vi "Test_RTC.vi"(8 "error in (no error)":errorcluster, 10 "Parameters":string, 11 "reference in":refnum<class "Test_Flux_Capacitor.lvclass">) -> (0 "error out":errorcluster, 2 "Result":bool, 3 "reference out":refnum<class "Test_Flux_Capacitor.lvclass">)   [LabVIEW 2022 SP3, in "Test_Flux_Capacitor.lvlib" / "Test_Flux_Capacitor.lvclass"]
uses:
  Test_Flux_Capacitor.lvclass
  ParameterTypes/RTC.ctl
  Components/SwitchBase.lvlibp/SwitchBase.lvclass
  Components/PSU_Base.lvlibp/PSU_Base.lvclass
  Components/Flux_Capacitor.lvlibp/Flux_Capacitor.lvclass
  <vilib>/JDP Science/JSONtext/JSONtext.lvlib
panel:
  in  "Parameter_Type":T1
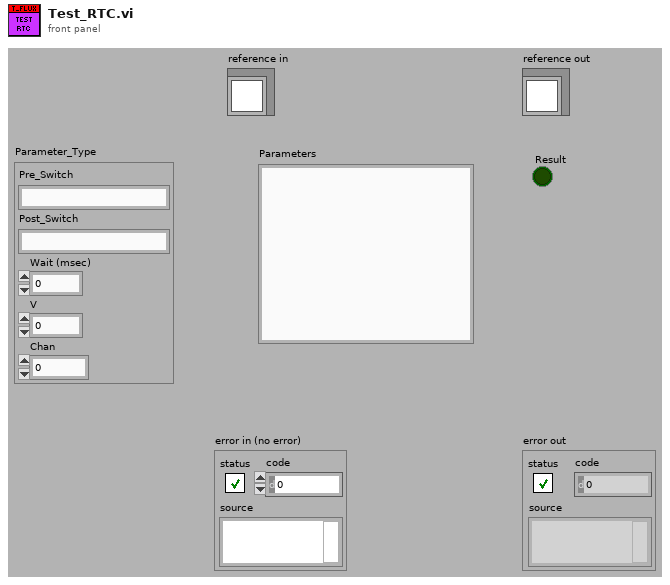
[diagram p1: front panel]
types:
  T1 = typedef "Test_Flux_Capacitor.lvlib/Test_Flux_Capacitor.lvclass/RTC.ctl" = cluster{"Pre_Switch":string, "Post_Switch":string, "Wait (msec)":u32, "V":dbl, "Chan":i32}
  T2 = typedef "Test_Flux_Capacitor.lvlib/Test_Flux_Capacitor.lvclass/ObjectAttributes.ctl" = cluster{"Config":T3, "DMM":refnum<class "DMM_Keysight_34980A.lvclass">, "LCR":refnum<class "LCR_BK891.lvclass">, "PSU":refnum<class "PSU_Base.lvclass">, "Switch_Manager":refnum<class "SwitchBase.lvclass">, "FRAM":string, "Flux_Capacitor":refnum<class "Flux_Capacitor.lvclass">, "Frequency_Counter":refnum<class "Frequency_Counter_Base.lvclass">, "JTAG":refnum<class "JTAG_Base.lvclass">}
  T3 = typedef "Test_Flux_Capacitor.lvlib/Test_Flux_Capacitor.lvclass/Config.ctl" = cluster{"default":string}
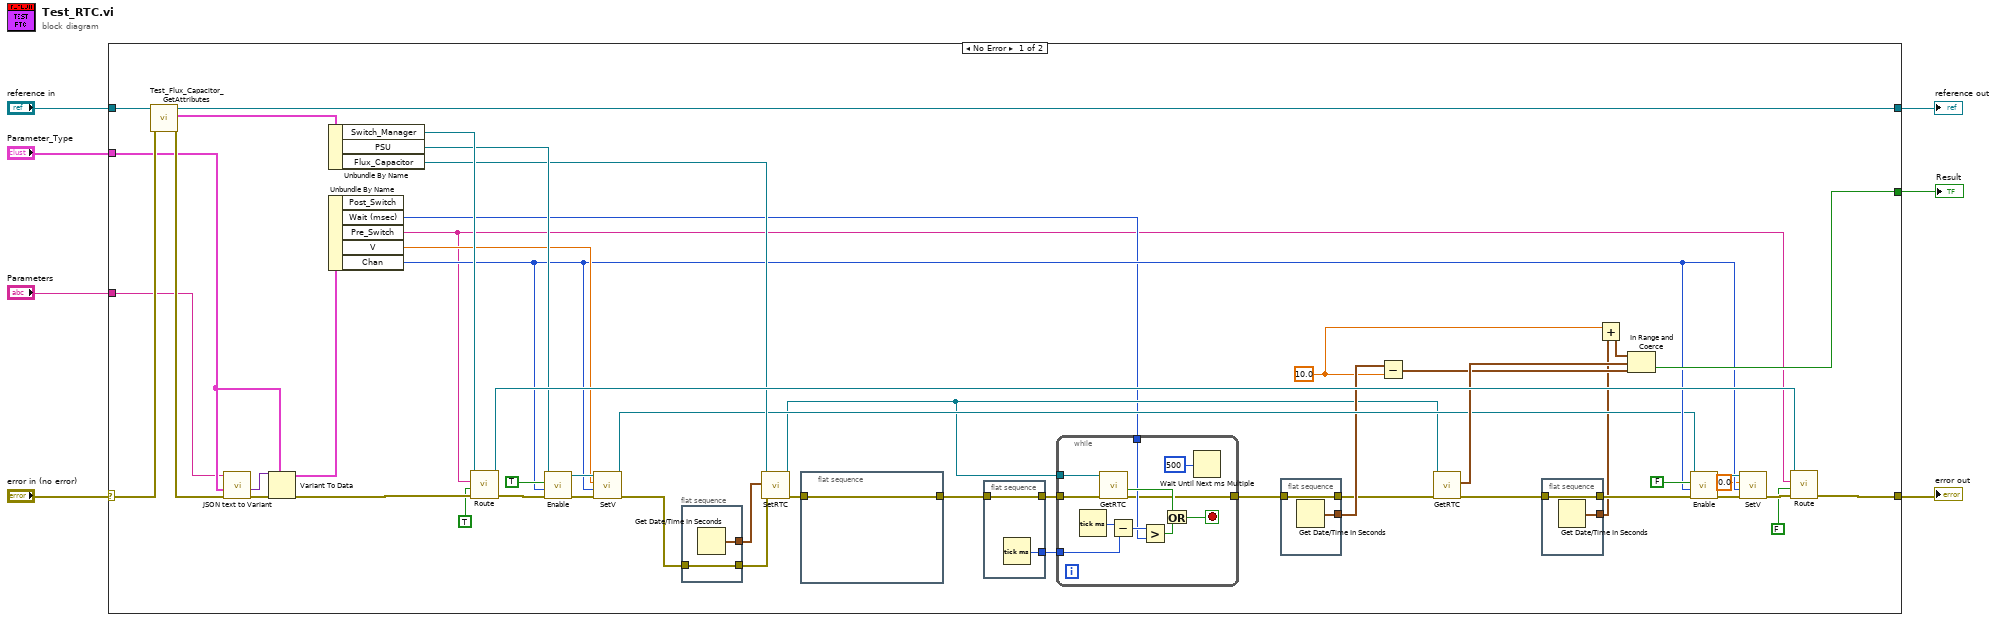
[diagram p0: block diagram]
diagram:
  n1 = case shown="No Error" "error in (no error)" {
    selector: "error in (no error)" -> [w58 w80]
    tunnel: [w51 w80] -> w6
    tunnel: [w56 w79] -> w4
    tunnel: "reference in" -> [w57 w79]
    tunnel: "Parameters" -> [w12 _]
    tunnel: "Parameter_Type" -> [w13 _]
    tunnel: [w38 _] -> w1
    frame No Error {
      w26 = 10.0
      n2 = call "Test_Flux_Capacitor_GetAttributes.vi"("error in (no error)"=w58, "reference in"=w57) -> ("error out"=w15:errorcluster, "Data"=w55:T2, "reference out"=w56:refnum<class "Test_Flux_Capacitor.lvclass">)  [unwired: 6 in, 1 out]
      n3 = call <vilib>:"JSON text to Variant.vi"("error in (no error)"=w15, "Data Type"=w13, "JSON"=w12) -> ("error out"=w14:errorcluster, "Variant out"=w11:variant)  [unwired: 7 in]
      n4 = Variant To Data(error in=w14, type=w13, Variant=w11) -> (data=w54:T1, error out=w50:errorcluster)
      n5 = Unbundle By Name(w55) -> ("Switch_Manager"=w53:refnum<class "SwitchBase.lvclass">, "PSU"=w47:refnum<class "PSU_Base.lvclass">, "Flux_Capacitor"=w43:refnum<class "Flux_Capacitor.lvclass">)
      n6 = Unbundle By Name(w54) -> ("Wait (msec)"=w16:u32, "Pre_Switch"=w9:string, "V"=w45:dbl, "Chan"=w31:i32)  [unwired: 1 out]
      n7 = call-dynamic "Route.vi"("error in (no error)"=w50, "Connect"=TRUE ("Enable"), "channel 1"=w9, "reference in"=w53) -> ("error out"=w49:errorcluster, "reference in"=w52:refnum<class "SwitchBase.lvclass">)  [unwired: 6 in]
      n8 = call-dynamic "Enable.vi"("error in (no error)"=w49, "Chan"=w31, "Enable"=TRUE, "reference in"=w47) -> ("error out"=w48:errorcluster, "reference in"=w46:refnum<class "PSU_Base.lvclass">)  [unwired: 6 in]
      n9 = call-dynamic "SetV.vi"("error in (no error)"=w48, "Chan"=w31, "V"=w45, "reference in"=w46) -> ("error out"=w32:errorcluster, "reference in"=w30:refnum<class "PSU_Base.lvclass">)  [unwired: 6 in]
      n10 = flat-sequence {
        tunnel: w32 -> [w78]
        tunnel: [w78] -> w42
        tunnel: [w77] -> w41
        frame #0 {
          n11 = Get Date/Time In Seconds() -> (seconds since 1Jan1904=w77:timestamp)
        }
      }
      n12 = call-dynamic "SetRTC.vi"("error in (no error)"=w42, "RTC"=w41, "reference in"=w43) -> ("error out"=w40:errorcluster, "reference in"=w20:refnum<class "Flux_Capacitor.lvclass">)  [unwired: 6 in, 1 out]
      n13 = flat-sequence {
        tunnel: w40 -> [w76]
        tunnel: [w76] -> w19
        frame #0 {
        }
      }
      n14 = flat-sequence {
        tunnel: w19 -> [w60]
        tunnel: [w60] -> w18
        tunnel: [w59] -> w17
        frame #0 {
          n15 = Tick Count (ms)() -> (millisecond timer value=w59:u32)
        }
      }
      n16 = while {
        tunnel: w18 -> [w70]
        tunnel: [w61] -> w21
        tunnel: w20 -> [w71]
        tunnel: w17 -> [w68]
        tunnel: w16 -> [w62]
        stop <- w64 stop-if-true
        n17 = Tick Count (ms)() -> (millisecond timer value=w69:u32)
        n18 = call-dynamic "GetRTC.vi"("error in (no error)"=w70, "reference in"=w71) -> ("error out"=w61:errorcluster, "OK"=w66:bool)  [unwired: 6 in, 2 out]
        n19 = Subtract(x=w69, y=w68) -> (x-y=w67:u32)
        n20 = Greater?(x=w67, y=w62) -> (0:w65:bool)
        n21 = Or(x=w66, y=w65) -> (x .or. y?=w64:bool)
        n22 = Wait Until Next ms Multiple(millisecond multiple=u32 500) -> ()  [unwired: 1 out]
      }
      n23 = flat-sequence {
        tunnel: [w75] -> w28
        tunnel: w21 -> [w74]
        tunnel: [w74] -> w22
        frame #0 {
          n24 = Get Date/Time In Seconds() -> (seconds since 1Jan1904=w75:timestamp)
        }
      }
      n25 = Subtract(x=w28, y=w26) -> (x-y=w27:timestamp)
      n26 = call-dynamic "GetRTC.vi"("error in (no error)"=w22, "reference in"=w20) -> ("error out"=w23:errorcluster, "RTC"=w39:timestamp)  [unwired: 6 in, 2 out]
      n27 = flat-sequence {
        tunnel: [w73] -> w25
        tunnel: w23 -> [w72]
        tunnel: [w72] -> w33
        frame #0 {
          n28 = Get Date/Time In Seconds() -> (seconds since 1Jan1904=w73:timestamp)
        }
      }
      n29 = Add(x=w26, y=w25) -> (x+y=w24:timestamp)
      n30 = In Range and Coerce(upper limit=w24, x=w39, lower limit=w27) -> (In Range?=w38:bool)  [unwired: 1 out]
      n31 = call-dynamic "Enable.vi"("error in (no error)"=w33, "Chan"=w31, "Enable"=FALSE, "reference in"=w30) -> ("error out"=w37:errorcluster, "reference in"=w36:refnum<class "PSU_Base.lvclass">)  [unwired: 6 in]
      n32 = call-dynamic "SetV.vi"("error in (no error)"=w37, "Chan"=w31, "V"=0.0, "reference in"=w36) -> ("error out"=w34:errorcluster)  [unwired: 6 in, 1 out]
      n33 = call-dynamic "Route.vi"("error in (no error)"=w34, "Connect"=FALSE ("Enable"), "channel 1"=w9, "reference in"=w52) -> ("error out"=w51:errorcluster)  [unwired: 6 in, 1 out]
    }
    frame Error {
    }
  }
  "Result" <- w1
  "error out" <- w6
  "reference out" <- w4
